vi "Q1.vi"() -> ()   [LabVIEW 2019]
uses:
  <vilib>/Utility/file.llb/Read From Spreadsheet File (DBL).vi
  <vilib>/measure/matone.llb/Extract Multiple Tone Information N Chan.vi
  <vilib>/measure/NI_MAPro.lvlib
panel:
  in  "ON\n\n\n\nOFF":bool
  out "multiple tone information":T1(array[cluster]) {"multiple tone information"."detected phase (deg)" format="%_6g"; "multiple tone information"."detected amplitude" format="%_6p"; "multiple tone information"."detected frequency frequency" format="%_6p"}
  out "Waveform Graph 2":waveform(dbl)[](graph)
  in  "Entrar agora com o novo arquivo tdms":path
  in  "Entrar com o arquivo txt original":path
  out "Data":dbl[][](array[numeric]) format="%0.3f"
  # "Esse arquivo segue os seguintes passos:\n1- Entrar com o arquivo .txt original;\n2- Esse arquivo será transformado em .tdms, então, você deve escolher o nome que deseja colocar no .tdms criado, juntamente com o local onde ele será salvo;\n3- O gráfico é gerado.\nOBS: Caso não dê certo, então repita o processo clicando sobre o arquivo .tdms exato que você havia criado antes. Então dará certo."
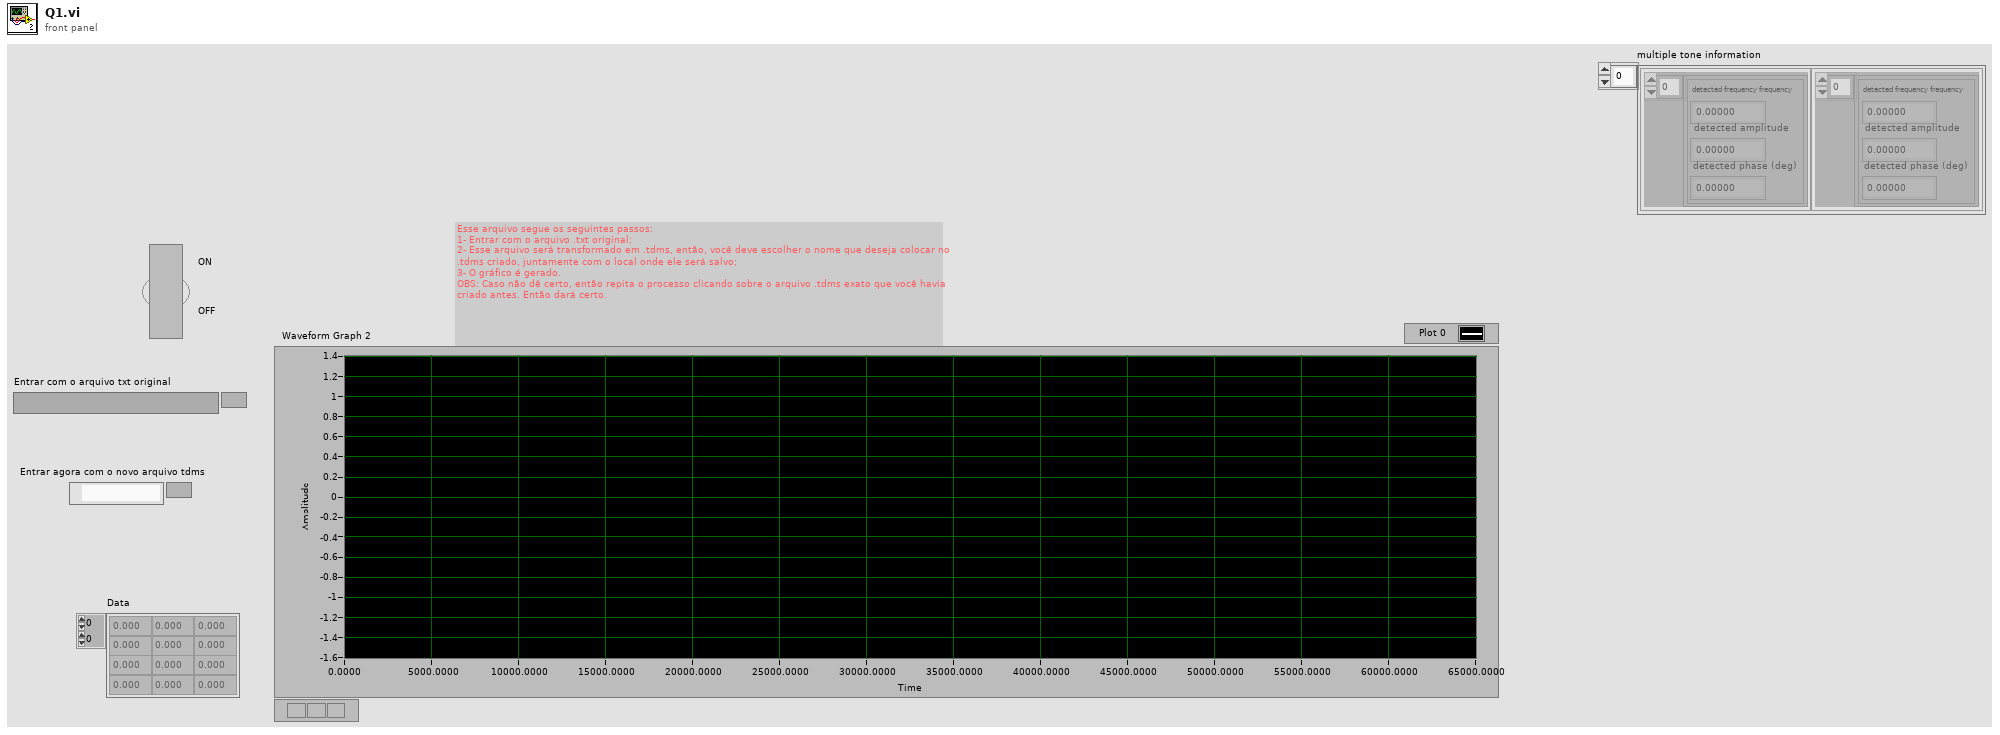
[diagram p1: front panel]
types:
  T1 = cluster{"multiple tone information":cluster{"detected frequency frequency":dbl, "detected amplitude":dbl, "detected phase (deg)":dbl}[]}[]
  T2 = enum16{"open", "open or create", "create or replace", "create", "open (read-only)"}
  T3 = cluster{"multiple tone information":cluster{"detected frequency":dbl, "detected amplitude":dbl, "detected phase (deg)":dbl}[]}[]
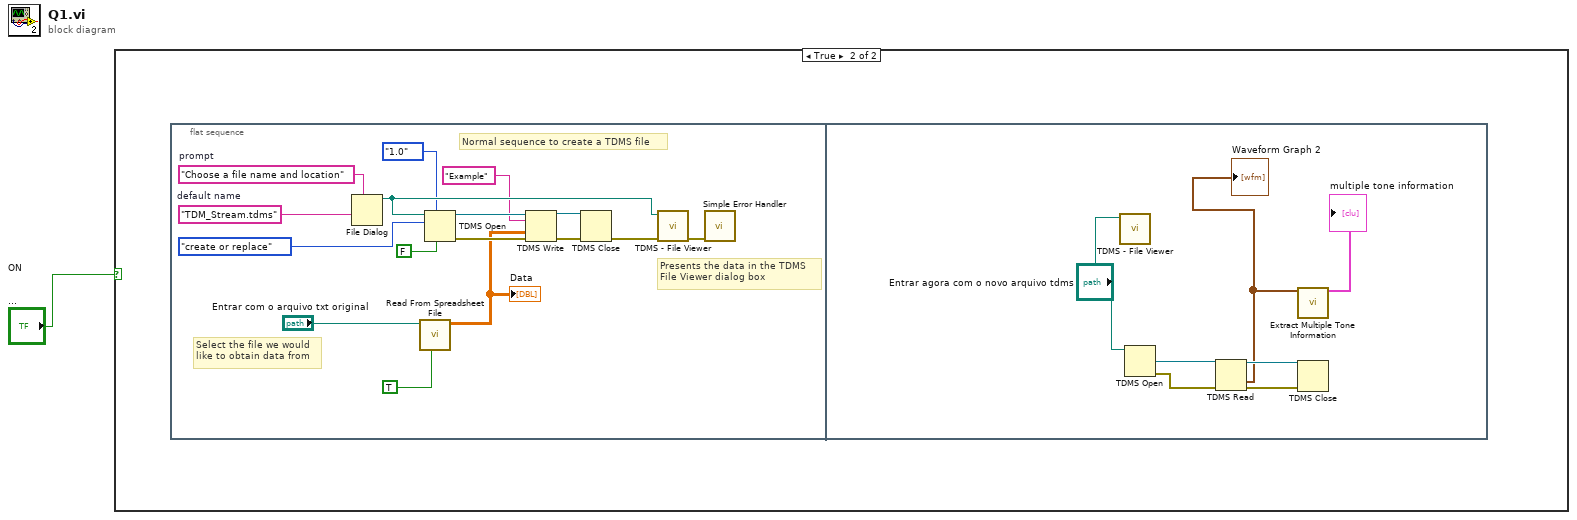
[diagram p0: block diagram]
diagram:
  n1 = case shown="True" "ON\n\n\n\nOFF" {
    frame False {
    }
    frame True {
      n2 = flat-sequence {
        frame #0 {
          w12 = "TDM_Stream.tdms"  # default name
          w13 = "Choose a file name and location"  # prompt
          # "Normal sequence to create a TDMS file"
          # "Presents the data in the TDMS \nFile Viewer dialog box"
          # "Select the file we would\nlike to obtain data from"
          n3 = File Dialog(7:w13, 9:w12) -> (3:w8:path)  [unwired: 1 in, 7 out]
          n4 = call-poly <vilib>:"Read From Spreadsheet File.vi"("transpose (no:F)"=TRUE, "file path (dialog if empty)"="Entrar com o arquivo txt original") -> ("all rows"=w3:dbl[][])  [unwired: 5 in, 4 out]
          "Data" <- w3
          n5 = TDMS Open(6:FALSE ("disable buffering (T)"), 7:enum16{"1.0", "2.0"}."1.0" ("file format version (2.0)"), 10:T2."create or replace" ("operation"), 11:w8) -> (0:w9:errorcluster, 3:w10:refnum<k34>)  [unwired: 3 in]
          n6 = TDMS Write(0:w10, 5:"Example" ("group name in (Untitled)"), 9:w3, 11:w9) -> (4:w17:refnum<k34>, 15:w14:errorcluster)  [unwired: 2 in, 2 out]
          n7 = TDMS Close(8:w14, 11:w17) -> (0:w16:errorcluster)  [unwired: 1 out]
          n8 = call <vilib>:"TDMS - File Viewer.vi"("error in (no error)"=w16, "file path"=w8) -> ("error out"=w15:errorcluster)  [unwired: 5 out]
          n9 = call <vilib>:"Simple Error Handler.vi"("error in (no error)"=w15) -> ()  [unwired: 1 in, 8 out]
        }
        frame #1 {
          n10 = call <vilib>:"TDMS - File Viewer.vi"("file path"="Entrar agora com o novo arquivo tdms") -> ()  [unwired: 5 in, 2 out]
          n11 = TDMS Open(11:"Entrar agora com o novo arquivo tdms") -> (0:w24:errorcluster, 3:w21:refnum<k34>)  [unwired: 6 in]
          n12 = TDMS Read(0:w21, 11:w24) -> (4:w23:refnum<k34>, 10:w19:waveform(dbl)[], 15:w22:errorcluster)  [unwired: 6 in, 3 out]
          "Waveform Graph 2" <- w19
          n13 = call-poly <vilib>:"Extract Multiple Tone Information.vi"("time signals in"=w19) -> ("multiple tone information"=→"multiple tone information":T3)  [unwired: 12 in, 2 out]
          n14 = TDMS Close(8:w22, 11:w23) -> ()  [unwired: 2 out]
        }
      }
    }
  }
